vi "XML setApiTokenResponse.vi"(11 "Token":string) -> (3 "Formatted XML":string, 5 "Time to Translate":u32)   [LabVIEW 2011]
uses:
  Controls/PIM.API.TOKEN.RESPONSE.ctl
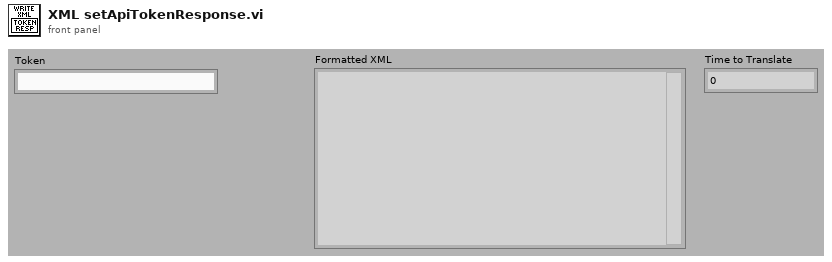
[diagram p1: front panel]
types:
  T1 = typedef "PIM.API.TOKEN.RESPONSE.ctl" = cluster{"#attributes":cluster{"xmlns":string, "xmlns:xsi":string, "xsi:schemaLocation":string}, "Token":string}
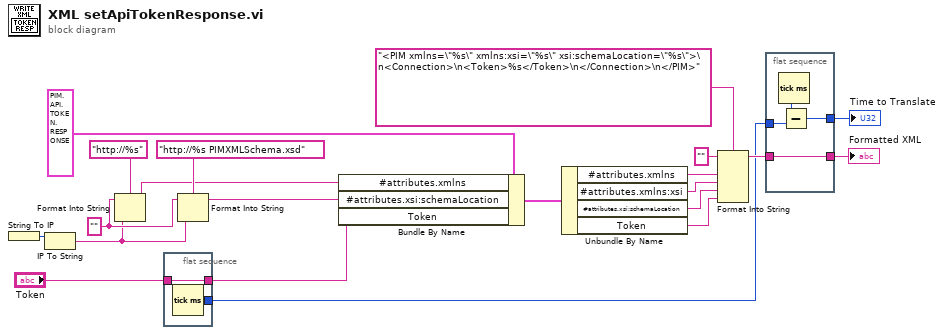
[diagram p0: block diagram]
diagram:
  w8 = "" ("initial string")
  n1 = String To IP() -> (0:w11:u32)  [unwired: 1 in]
  n2 = IP To String(2:w11) -> (0:w7:string)  [unwired: 1 in]
  n3 = Format Into String(format string="http://%s" ("xmlns"), initial string=w8, w7) -> (resulting string=w6:string)  [unwired: 1 in, 1 out]
  n4 = flat-sequence {
    tunnel: [w23] -> w15
    tunnel: "Token" -> [w22]
    tunnel: [w22] -> w1
    frame #0 {
      n5 = Tick Count (ms)() -> (millisecond timer value=w23:u32)
    }
  }
  n6 = Format Into String(format string="http://%s PIMXMLSchema.xsd" ("xsi:schemaLocation"), initial string=w8, w7) -> (resulting string=w5:string)  [unwired: 1 in, 1 out]
  n7 = Bundle By Name(cluster=T1 {"#attributes"={"xmlns"="http://www.kaelus.com", "xmlns:xsi"="http://www.w3.org/2001/XMLSchema-instance", "xsi:schemaLocation"="http://www.kaelus.com PIMXMLSchema.xsd"}, "Token"=""} ("PIM"), "#attributes.xmlns"=w6, "#attributes.xsi:schemaLocation"=w5, "Token"=w1) -> (w3:T1)
  n8 = Unbundle By Name(w3) -> ("#attributes.xmlns"=w20:string, "#attributes.xmlns:xsi"=w19:string, "#attributes.xsi:schemaLocation"=w18:string, "Token"=w13:string)
  n9 = Format Into String(format string="<PIM xmlns=\"%s\" xmlns:xsi=\"%s\" xsi:schemaLocation=\"%s\">\n<Connection>\n<Token>%s</Token>\n</Connection>\n</PIM>", initial string="", w20, w19, w18, w13) -> (resulting string=w17:string)  [unwired: 1 in, 1 out]
  n10 = flat-sequence {
    tunnel: w17 -> [w27]
    tunnel: [w27] -> w16
    tunnel: w15 -> [w26]
    tunnel: [w24] -> w14
    frame #0 {
      n11 = Tick Count (ms)() -> (millisecond timer value=w25:u32)
      n12 = Subtract(x=w25, y=w26) -> (x-y=w24:u32)
    }
  }
  "Formatted XML" <- w16
  "Time to Translate" <- w14
